vi "Utility_Read_Refrigerant_File.vi"(6 "error in (no error)":errorcluster, 8 "Refprop Main Directory":path, 9 "Refrigerant File":string) -> (0 "error out":errorcluster, 3 "Mixure Cluster":T1)   [LabVIEW 2016]
doc: "Reads a refrigerant file and outputs a cluster of mixture properties \n\nDeveloped by:\nGreg Sussman\nProcess Automation Corp\nwww.processauto.com\n(267)685-1249"
uses:
  Ctl/Mixture Composition cluster_d.ctl
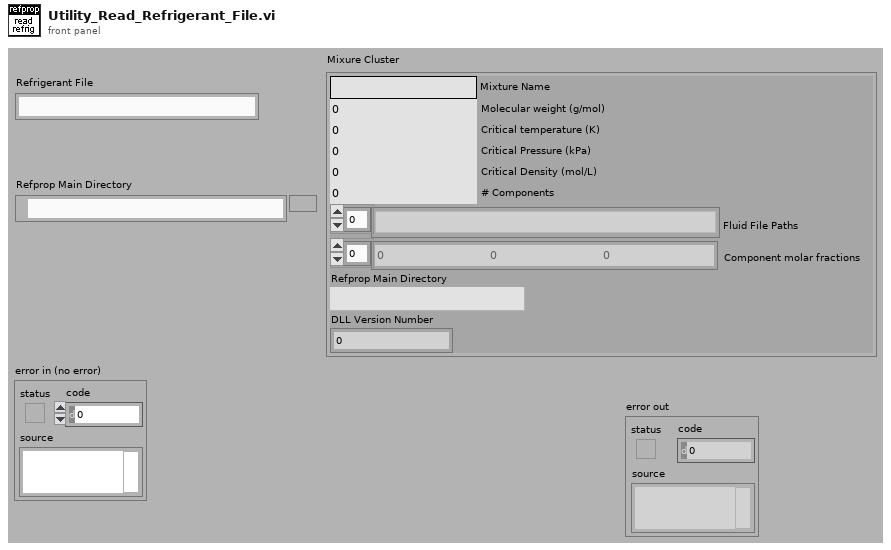
[diagram p1: front panel]
types:
  T1 = typedef "Mixture Composition cluster_d.ctl" = cluster{"Mixture Name":string, "Molecular weight (g/mol)":dbl, "Critical temperature (K)":dbl, "Critical Pressure (kPa)":dbl, "Critical Density (mol/L)":dbl, "# Components":i32, "Fluid File Paths":path[], "Component molar fractions":dbl[], "Refprop Main Directory":path, "DLL Version Number":dbl}
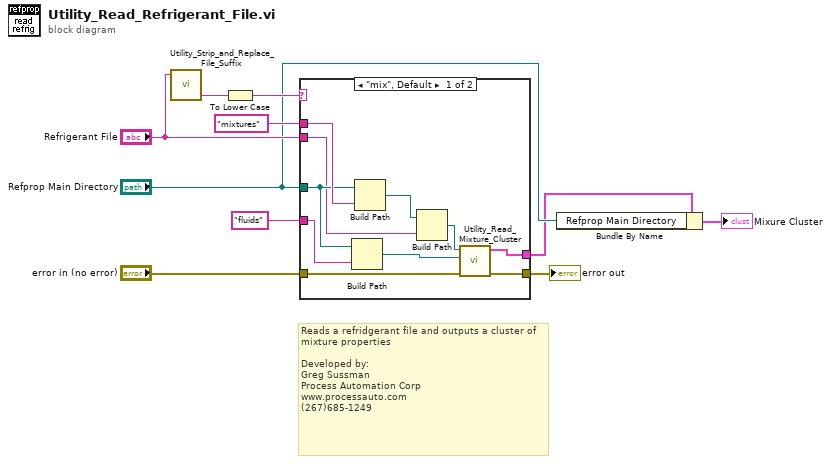
[diagram p0: block diagram]
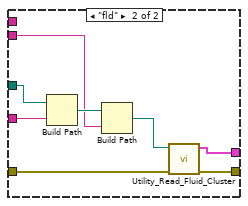
[diagram p2: hidden frame]
diagram:
  # "Reads a refridgerant file and outputs a cluster of mixture properties \n\nDeveloped by:\nGreg Sussman\nProcess Automation Corp\nwww.processauto.com\n(267)685-1249"
  n1 = call "Utility_Strip_and_Replace_File_Suffix.vi"("File Name"="Refrigerant File") -> ("Old File Suffix OUT"=w7:string)  [unwired: 3 in, 1 out]
  n2 = To Lower Case(string=w7) -> (all lower case string=w10:string)
  n3 = case shown="\"mix\", Default" w10 {
    tunnel: "Refprop Main Directory" -> [w15 w25]
    tunnel: [w11 w21] -> w2
    tunnel: "error in (no error)" -> [w20 w28]
    tunnel: [w19 w27] -> w8
    tunnel: "fluids" -> [w16 w26]
    tunnel: "Refrigerant File" -> [w13 w23]
    tunnel: "mixtures" -> [w18 _]
    frame "mix", Default {
      n4 = Build Path(base path=w15, name or relative path=w16) -> (appended path=w14:path)
      n5 = Build Path(base path=w15, name or relative path=w18) -> (appended path=w17:path)
      n6 = Build Path(base path=w17, name or relative path=w13) -> (appended path=w12:path)
      n7 = call "Utility_Read_Mixture_Cluster.vi"("error in (no error)"=w20, "Dir containing fluid files"=w14, "Mixture File"=w12) -> ("error out"=w19:errorcluster, "Mixure Cluster"=w11:T1)  [unwired: 5 in]
    }
    frame "fld" {
      n8 = Build Path(base path=w25, name or relative path=w26) -> (appended path=w24:path)
      n9 = Build Path(base path=w24, name or relative path=w23) -> (appended path=w22:path)
      n10 = call "Utility_Read_Fluid_Cluster.vi"("error in (no error)"=w28, "Fluid File"=w22) -> ("error out"=w27:errorcluster, "Fluid Cluster"=w21:T1)  [unwired: 6 in]
    }
  }
  "error out" <- w8
  n11 = Bundle By Name(cluster=w2, "Refprop Main Directory"="Refprop Main Directory") -> (→"Mixure Cluster":T1)
